vi "Stop Work.vi"(6 "Controller name":string, 8 "error in (no error)":errorcluster, 9 "Reply":bool=TRUE, 10 "Reply to":refnum<class "Stop Response Msg.lvclass">, 11 "Measure Object in":refnum<class "Process Object.lvclass">) -> (0 "error out":errorcluster, 3 "Measure Object out":refnum<class "Process Object.lvclass">)   [LabVIEW 2021, in "Process Object.lvclass"]
uses:
  Process Object.lvclass
  C:/Program Files/National Instruments/LabVIEW 2021/vi.lib/ActorFramework/Actor/Actor.lvclass
  Controllers/Process Controller Messages/Stop Response Msg/Stop Response Msg.lvclass
  <vilib>/ActorFramework/Actor/Actor.lvclass/Actor.ctl
  <vilib>/ActorFramework/Message Enqueuer/Message Enqueuer.lvclass/Message Enqueuer.ctl
  Publish-Subscribe/Interfaces/Publisher Messages/Unsubscribe Msg/Unsubscribe Msg.lvclass/Unsubscribe Msg.ctl
  <vilib>/ActorFramework/Message Enqueuer/Init from Existing Queue.vi
  <vilib>/ActorFramework/Message Enqueuer/Enqueue.vi
  Publish-Subscribe/Interfaces/Publisher Messages/Unsubscribe Msg/Unsubscribe Msg.lvclass
  C:/Program Files/National Instruments/LabVIEW 2021/vi.lib/ActorFramework/Message/Message.lvclass
  <vilib>/ActorFramework/Message Priority Queue/Priority Enqueue.vi
  Worker/Worker Actor/Worker Actor.lvclass
  <vilib>/ActorFramework/Message Enqueuer/Message Enqueuer.lvclass
  Process Object.lvclass/Process Object.ctl
  <vilib>/ActorFramework/Actor/Actor.lvclass
  C:/GitHub/LabActor/Worker/Worker Actor/Worker Actor.lvclass
  C:/GitHub/LabActor/Template Module/Template Module.lvclass
  C:/GitHub/LabActor/Worker/Woker Interface/Worker.lvclass
  C:/GitHub/LabActor/Process Object/Process Object.lvclass
  C:/GitHub/LabActor/Publish-Subscribe/Interfaces/Subscriber/Subscriber.lvclass
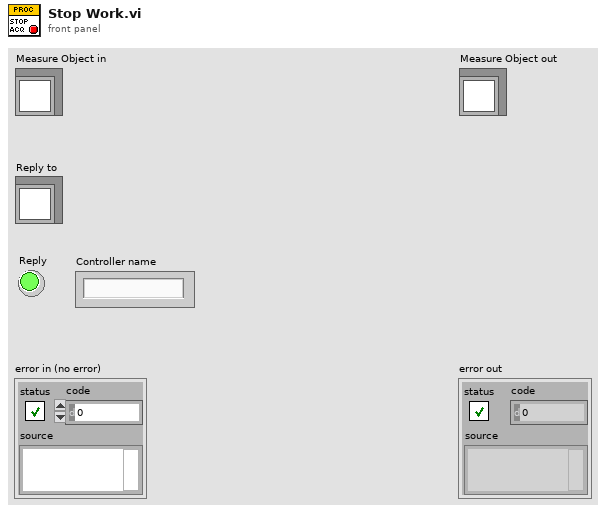
[diagram p1: front panel]
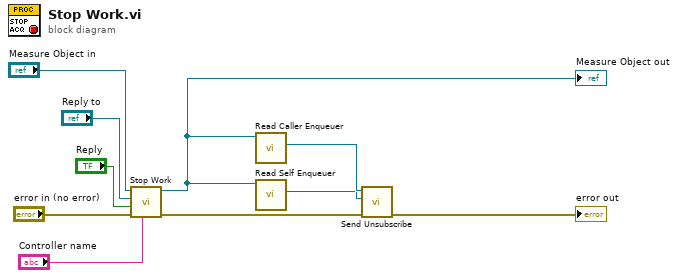
[diagram p0: block diagram]
diagram:
  n1 = call-parent "Stop Work.vi"("Controller name"="Controller name", "error in (no error)"="error in (no error)", "Reply"="Reply", "Reply to"="Reply to", "Measure Object in"="Measure Object in") -> ("error out"=w5:errorcluster, "Measure Object out"=w6:refnum<class "Process Object.lvclass">)  [unwired: 5 in]
  "Measure Object out" <- w6
  n2 = call <vilib>:"Read Caller Enqueuer.vi"("Actor"=w6) -> ("Caller Enqueuer"=w2:refnum<class "Message Enqueuer.lvclass">)  [unwired: 10 in]
  n3 = call <vilib>:"Read Self Enqueuer.vi"("Actor"=w6) -> ("Self Enqueuer"=w1:refnum<class "Message Enqueuer.lvclass">)  [unwired: 10 in]
  n4 = call "Send Unsubscribe.vi"("error in (no error)"=w5, "Subscriber Enq"=w1, "Message Enqueuer"=w2) -> ("error out"=→"error out":errorcluster)  [unwired: 7 in, 1 out]
